vi "Lift Teleop Call.vi"(10 "Button Values":bool[](array[boolean])) -> ()   [LabVIEW 2017]
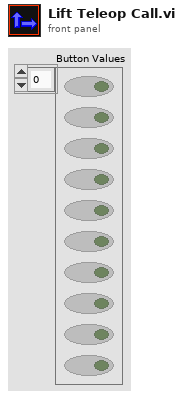
[diagram p1: front panel]
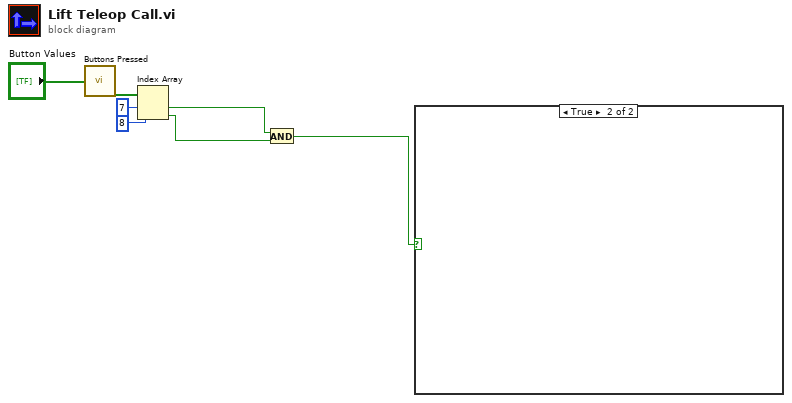
[diagram p0: block diagram]
diagram:
  n1 = call "Buttons Pressed.vi"("Button Values"="Button Values") -> ("Button Presses"=w7:bool[])
  n2 = Index Array(array=w7, index #1=7 ("index"), index #2=8 ("index")) -> (element #1=w3:bool, element #2=w2:bool)
  n3 = And(x=w3, y=w2) -> (x .and. y?=w1:bool)
  n4 = case shown="True" w1 {
    frame False {
    }
    frame True {
    }
  }
